vi "copy plot colours and visibility.vi"(8 "error in":errorcluster, 10 "XY Graph (print)":refnum<vi>, 11 "XY Graph (main VI)":refnum<vi>) -> (0 "error out":errorcluster)   [LabVIEW 2014]
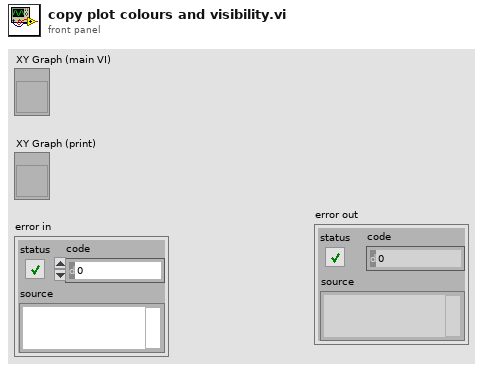
[diagram p1: front panel]
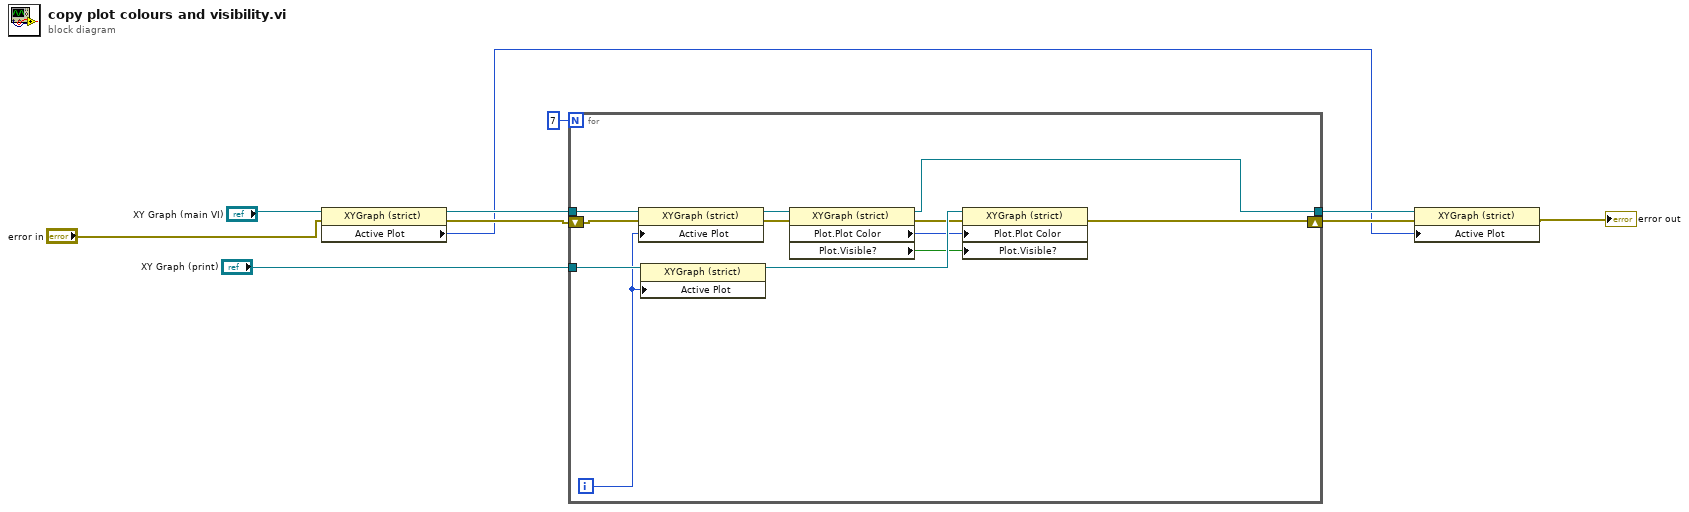
[diagram p0: block diagram]
diagram:
  n1 = property class="XYGraph (strict)"(reference="XY Graph (main VI)", error in="error in") -> (reference out=w9:refnum<vi>, error out=w8:errorcluster, "Active Plot"=w3:u32)
  n2 = for {
    N: 7 -> [_]
    shift-right: [w13] -> w4
    shift-left: w8 -> [w21]
    tunnel: "XY Graph (print)" -> [w20]
    tunnel: w9 -> [w22]
    tunnel: [w12] -> w5
    i -> [w19]
    n3 = property class="XYGraph (strict)"(reference=w22, error in=w21, "Active Plot"=w19) -> (reference out=w18:refnum<vi>, error out=w14:errorcluster)
    n4 = property class="XYGraph (strict)"(reference=w20, "Active Plot"=w19) -> (reference out=w17:refnum<vi>)  [unwired: 1 in, 1 out]
    n5 = property class="XYGraph (strict)"(reference=w18, error in=w14) -> (reference out=w12:refnum<vi>, error out=w15:errorcluster, "Plot.Plot Color"=w16:u32, "Plot.Visible?"=w11:bool)
    n6 = property class="XYGraph (strict)"(reference=w17, error in=w15, "Plot.Plot Color"=w16, "Plot.Visible?"=w11) -> (error out=w13:errorcluster)  [unwired: 1 out]
  }
  n7 = property class="XYGraph (strict)"(reference=w5, error in=w4, "Active Plot"=w3) -> (error out=→"error out":errorcluster)  [unwired: 1 out]
